vi "Draw Filled Triangle (Old).vi"(4 "Alpha":dbl, 7 "Enable Alpha Blending (F)":bool, 10 "Triangle":T1={"Vertex 1"={"Position"={"x"=0.0, "y"=0.0, "z"=0.0}, "UV"={"u"=0.0, "v"=0.0}, "Colour"=12517256}, "Vertex 2"={"Position"={"x"=0.0, "y"=0.0, "z"=0.0}, "UV"={"u"=0.0, "v"=0.0}, "Colour"=12517256}, "Vertex 3"={"Position"={"x"=0.0, "y"=0.0, "z"=0.0}, "UV"={"u"=0.0, "v"=0.0}, "Colour"=12517256}, "Colour"=0} {"Vertex 3"."UV"."v" min=0 max=1 step=0.1; "Vertex 3"."UV"."u" min=0 max=1 step=0.1; "Vertex 2"."UV"."v" min=0 max=1 step=0.1; "Vertex 2"."UV"."u" min=0 max=1 step=0.1; "Vertex 1"."UV"."v" min=0 max=1 step=0.1; "Vertex 1"."UV"."u" min=0 max=1 step=0.1}, 11 "Pixel Data in":u32[][](array[numeric])) -> (3 "Pixel Data out":u32[][](array[numeric]))   [LabVIEW 2020]
uses:
  Raster (FPGA).lvlib
  Method.ctl
  Point 2D (I32).ctl
  Vector 3D.ctl
  UV.ctl
  Vertex.ctl
  Triangle.ctl
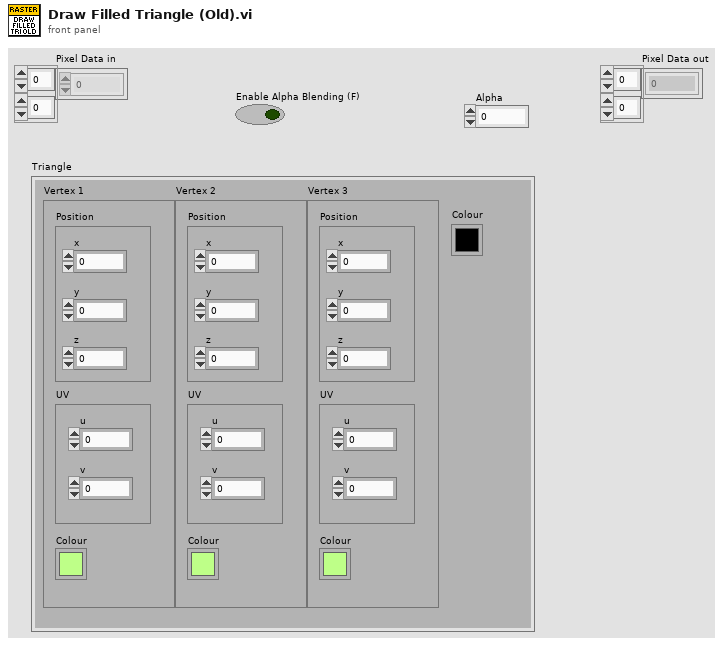
[diagram p1: front panel]
types:
  T1 = typedef "Raster (FPGA).lvlib/Triangle.ctl" = cluster{"Vertex 1":T2, "Vertex 2":T2, "Vertex 3":T2, "Colour":u32}
  T2 = typedef "Raster (FPGA).lvlib/Vertex.ctl" = cluster{"Position":T3, "UV":T4, "Colour":u32}
  T3 = typedef "Raster (FPGA).lvlib/Vector 3D.ctl" = cluster{"x":sgl, "y":sgl, "z":sgl}
  T4 = typedef "Raster (FPGA).lvlib/UV.ctl" = cluster{"u":sgl, "v":sgl}
  T5 = typedef "Raster (FPGA).lvlib/Triangle (Sorted).ctl" = cluster{"Top Vertex":T2, "Mid Vertex":T2, "Bottom Vertex":T2, "Colour":u32}
  T6 = typedef "Raster (FPGA).lvlib/Method.ctl" = enum16{"Per item", "Row", "Replace Array Subset", "MoveBlock", " MoveBlock2 "}
  T7 = typedef "Raster (FPGA).lvlib/Point 2D (I32).ctl" = cluster{"x":i32, "y":i32}
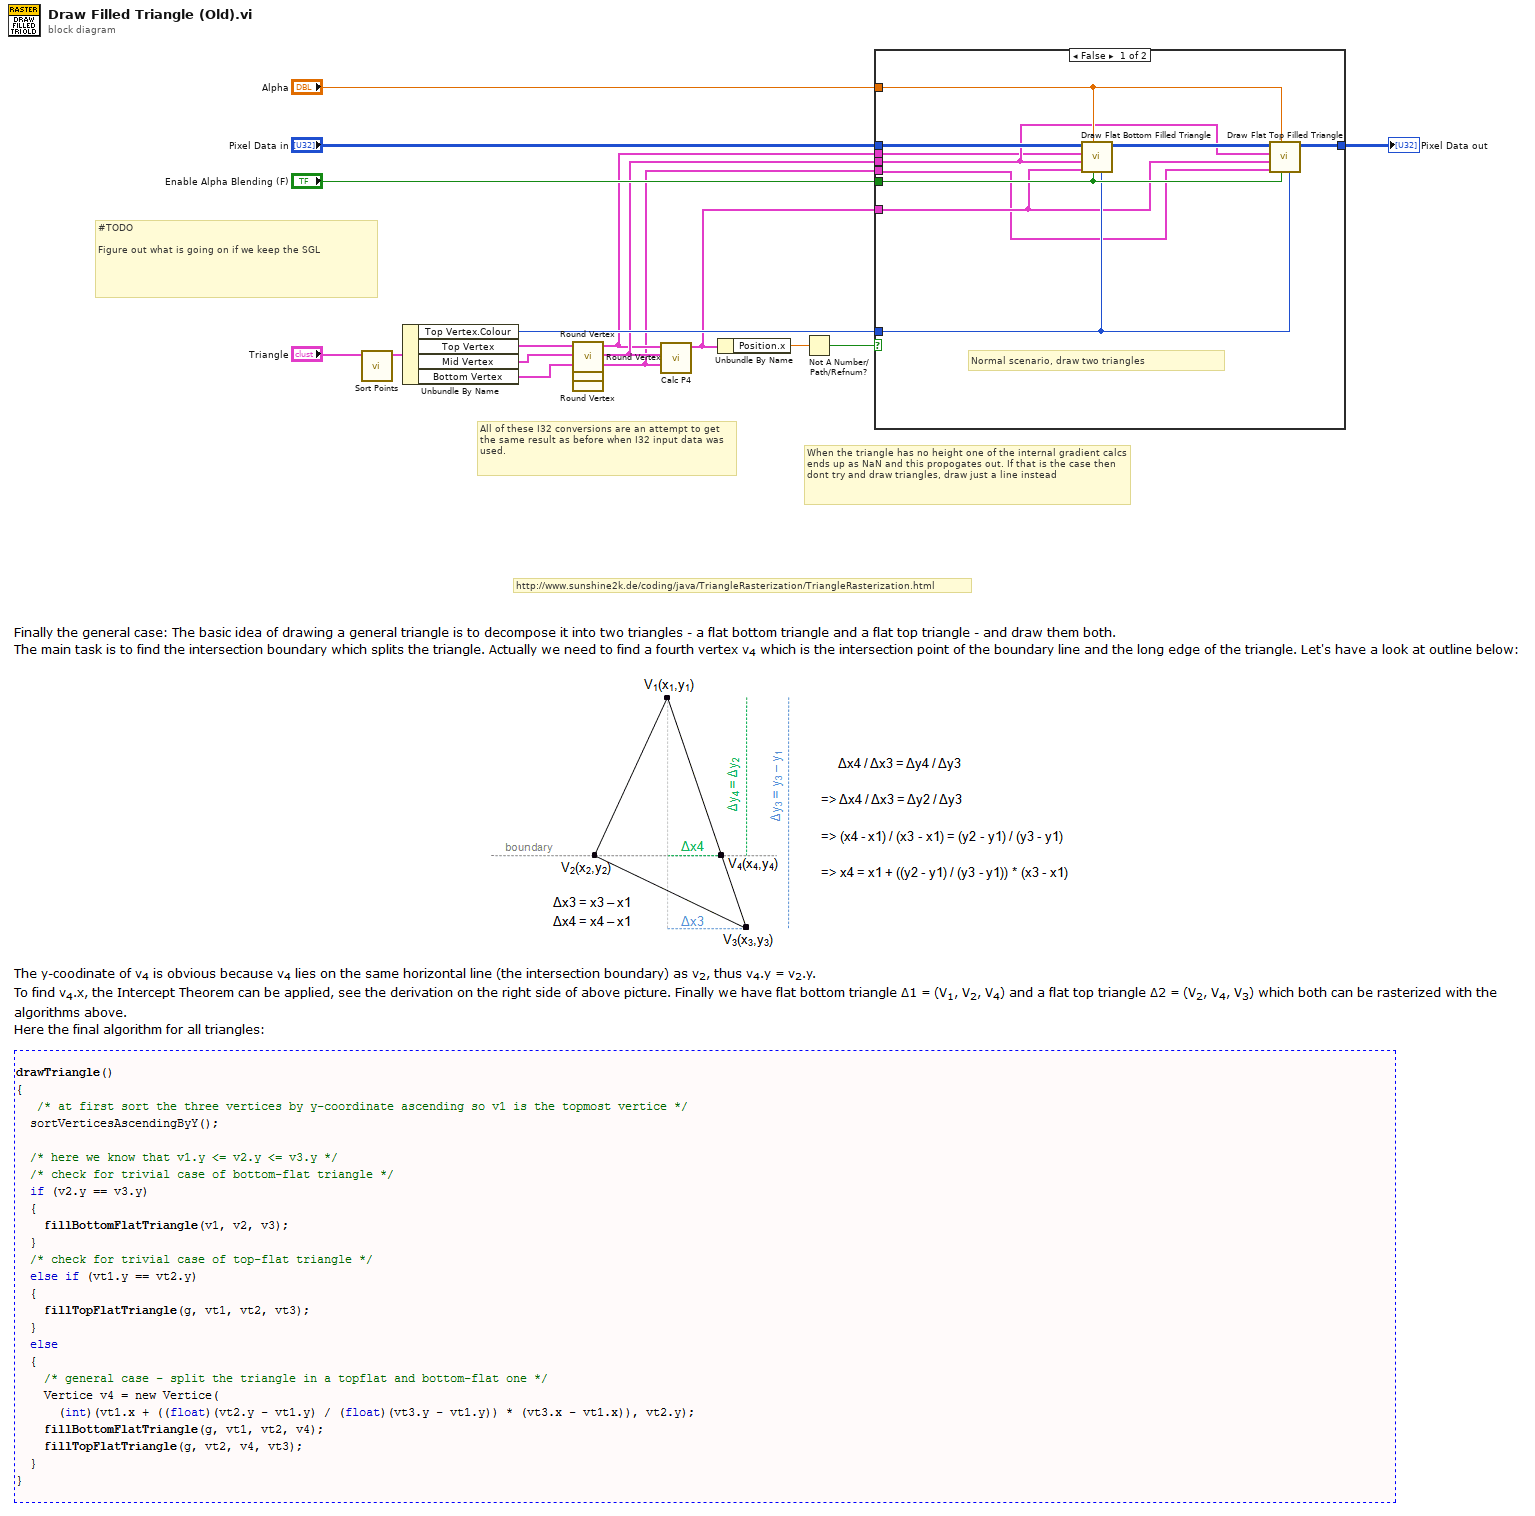
[diagram p0: block diagram]
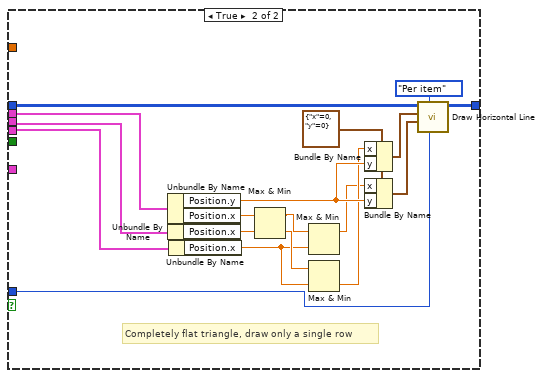
[diagram p2: hidden frame]
diagram:
  # "When the triangle has no height one of the internal gradient calcs ends up as NaN and this propogates out. If that is the case then dont try and draw triangles, draw just a line instead"
  # "#TODO\n\nFigure out what is going on if we keep the SGL"
  # "All of these I32 conversions are an attempt to get the same result as before when I32 input data was used."
  # "http://www.sunshine2k.de/coding/java/TriangleRasterization/TriangleRasterization.html"
  n1 = call "Sort Points.vi"("Triangle"="Triangle") -> ("Sorted Triangle"=w10:T5)  [unwired: 10 in]
  n2 = Unbundle By Name(w10) -> ("Top Vertex.Colour"=w11:u32, "Top Vertex"=w4:T2, "Mid Vertex"=w3:T2, "Bottom Vertex"=w2:T2)
  n3 = call "Round Vertex.vi"("Vertex in"=w4) -> ("Vertex With Position Rounded"=w5:T2)  [unwired: 10 in]
  n4 = call "Round Vertex.vi"("Vertex in"=w3) -> ("Vertex With Position Rounded"=w9:T2)  [unwired: 10 in]
  n5 = call "Round Vertex.vi"("Vertex in"=w2) -> ("Vertex With Position Rounded"=w1:T2)  [unwired: 10 in]
  n6 = call "Calc P4.vi"("Bottom"=w1, "Middle"=w9, "Top"=w5) -> ("Point 4"=w6:T2)  [unwired: 8 in]
  n7 = Unbundle By Name(w6) -> ("Position.x"=w8:sgl)
  n8 = Not A Number/Path/Refnum?(number/path/refnum=w8) -> (NaN/Path/Refnum?=w7:bool)
  n9 = case shown="False" w7 {
    tunnel: [w26 w44] -> w16
    tunnel: "Pixel Data in" -> [w25 w43]
    tunnel: "Enable Alpha Blending (F)" -> [w24 _]
    tunnel: "Alpha" -> [w23 _]
    tunnel: w11 -> [w22 w30]
    tunnel: w9 -> [w20 w28]
    tunnel: w5 -> [w19 w29]
    tunnel: w6 -> [w18 _]
    tunnel: w1 -> [w17 w27]
    frame False {
      # "Normal scenario, draw two triangles"
      n10 = call "Draw Flat Bottom Filled Triangle.vi"("Fill Colour"=w22, "Enable Alpha Blending (F)"=w24, "Alpha"=w23, "Vertex 3"=w18, "Vertex 2"=w20, "Vertex 1"=w19, "Pixel Data in"=w25) -> ("Pixel Data out"=w21:u32[][])  [unwired: 4 in]
      n11 = call "Draw Flat Top Filled Triangle.vi"("Fill Colour"=w22, "Enable Alpha Blending (F)"=w24, "Alpha"=w23, "Vertex 3"=w17, "Vertex 2"=w18, "Vertex 1"=w20, "Pixel Data in"=w21) -> ("Pixel Data out"=w26:u32[][])  [unwired: 4 in]
    }
    frame True {
      w36 = T7 {"x"=0, "y"=0} ("Point 1")
      # "Completely flat triangle, draw only a single row"
      n12 = Unbundle By Name(w29) -> ("Position.y"=w35:sgl, "Position.x"=w41:sgl)
      n13 = Unbundle By Name(w28) -> ("Position.x"=w40:sgl)
      n14 = Unbundle By Name(w27) -> ("Position.x"=w37:sgl)
      n15 = Max & Min(x=w41, y=w40) -> (max(x,y)=w39:sgl, min(x,y)=w38:sgl)
      n16 = Max & Min(x=w39, y=w37) -> (max(x,y)=w31:sgl)  [unwired: 1 out]
      n17 = Max & Min(x=w38, y=w37) -> (min(x,y)=w32:sgl)  [unwired: 1 out]
      n18 = Bundle By Name(cluster=w36, "x"=w32, "y"=w35) -> (w34:T7)
      n19 = Bundle By Name(cluster=w36, "x"=w31, "y"=w35) -> (w33:T7)
      n20 = call "Draw Horizontal Line.vi"("Colour"=w30, "Method"=Method."Per item", "Point 2"=w33, "Point 1"=w34, "Pixel Data in"=w43) -> ("Pixel Data out"=w44:u32[][])  [unwired: 6 in]
    }
  }
  "Pixel Data out" <- w16
